vi "Do.vi"(8 "Error In":errorcluster, 10 "Actor in":refnum<class "Actor.lvclass">, 11 "LNA Return Message Msg":refnum<class "LNA Return Message Msg.lvclass">) -> (0 "Error Out":errorcluster, 2 "Actor out":refnum<class "Actor.lvclass">)   [LabVIEW 2014, in "CS++RTMain.lvlib" / "LNA Return Message Msg.lvclass"]
doc: "(<B>Filename</B>: Actor Framework.lvlib:Message.lvclass:Do.vi)\n\nDefines what a message does when it is received by an actor. Generally, a message instructs an actor to invoke one of its methods. By default, this method does nothing. A child class must override it to define behavior. Create a child class by using the Actor Framework Message Maker dialog box."
uses:
  LNA Return Message Msg.lvclass
  <vilib>/ActorFramework/Actor/Actor.lvclass
  <vilib>/NI/Actors/Linked Network Actor/Linked Network Actor Messages/LNA Return Message Msg/LNA Return Message Msg.lvclass
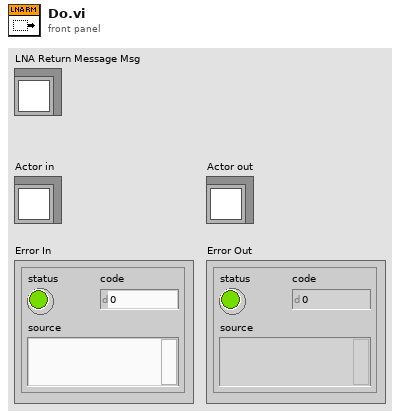
[diagram p1: front panel]
types:
  T1 = typedef "Actor Framework.lvlib/Message Enqueuer.lvclass/Message Priority.ctl" = enum16{"Low", "Normal", "High"}
  T2 = cluster{"Tx Message":refnum<class "Message.lvclass">, "Tx Error":errorcluster, "Message Priority":T1}
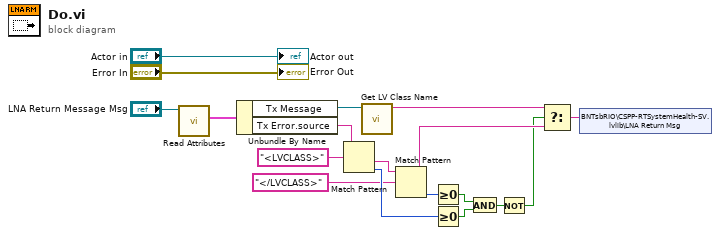
[diagram p0: block diagram]
diagram:
  n1 = call <vilib>:"Read Attributes.vi"("Abstract Message Template in"="LNA Return Message Msg") -> ("Payload"=w15:T2)  [unwired: 9 in, 1 out]
  n2 = Unbundle By Name(w15) -> ("Tx Message"=w14:refnum<class "Message.lvclass">, "Tx Error.source"=w6:string)
  n3 = Match Pattern(string=w6, regular expression="<LVCLASS>" ("string")) -> (after substring=w7:string, offset past match=w10:i32)  [unwired: 1 in, 2 out]
  n4 = call <vilib>:"Get LV Class Name.vi"("object"=w14) -> ("class name"=w4:string)  [unwired: 9 in, 1 out]
  n5 = Match Pattern(string=w7, regular expression="</LVCLASS>" ("string")) -> (before substring=w3:string, offset past match=w11:i32)  [unwired: 1 in, 2 out]
  n6 = Greater Or Equal To 0?(x=w11) -> (x >= 0?=w12:bool)
  n7 = Greater Or Equal To 0?(x=w10) -> (x >= 0?=w13:bool)
  n8 = And(x=w12, y=w13) -> (x .and. y?=w5:bool)
  n9 = Not(x=w5) -> (.not. x?=w2:bool)
  n10 = Select(t=w4, s=w2, f=w3) -> (s? t:f=w1:string)
  n11 = shared-variable "BNTsbRIO\\CSPP-RTSystemHealth-SV.lvlib\\LNA Return Msg"(w1) -> ()  [unwired: 1 in, 1 out]
  "Error Out" <- "Error In"
  "Actor out" <- "Actor in"
